vi "PacketToBuffer.vi"(11 "Packet":T1) -> (3 "Data":u8[](array[numeric]))   [LabVIEW 2009]
uses:
  Packet.ctl
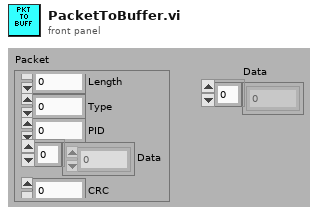
[diagram p1: front panel]
types:
  T1 = typedef "Packet.ctl" = cluster{"Length":u8, "Type":u8, "PID":u8, "Data":u8[], "CRC":u8}
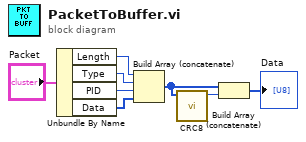
[diagram p0: block diagram]
diagram:
  n1 = Unbundle By Name("Packet") -> ("Length"=w7:u8, "Type"=w6:u8, "PID"=w5:u8, "Data"=w4:u8[])
  n2 = Build Array (concatenate)(w7, w6, w5, w4) -> (w3:u8[])
  n3 = call "CRC8.vi"("Data"=w3) -> ("CRC8"=w2:u8)  [unwired: 10 in]
  n4 = Build Array (concatenate)(w3, w2) -> (→"Data":u8[])
